vi "PIC1_DEMO.vi"() -> ()   [LabVIEW 2016]
uses:
  <vilib>/picture/picture.llb/imagedata.ctl
panel:
  out "image":u8[](array[numeric]) format="%x"
  out "size(s)":i32[](array[numeric])
  out "24-bit pixmap":u32[][](array[numeric]) format="%x"
  out "image data":T1
  out "new picture":picture
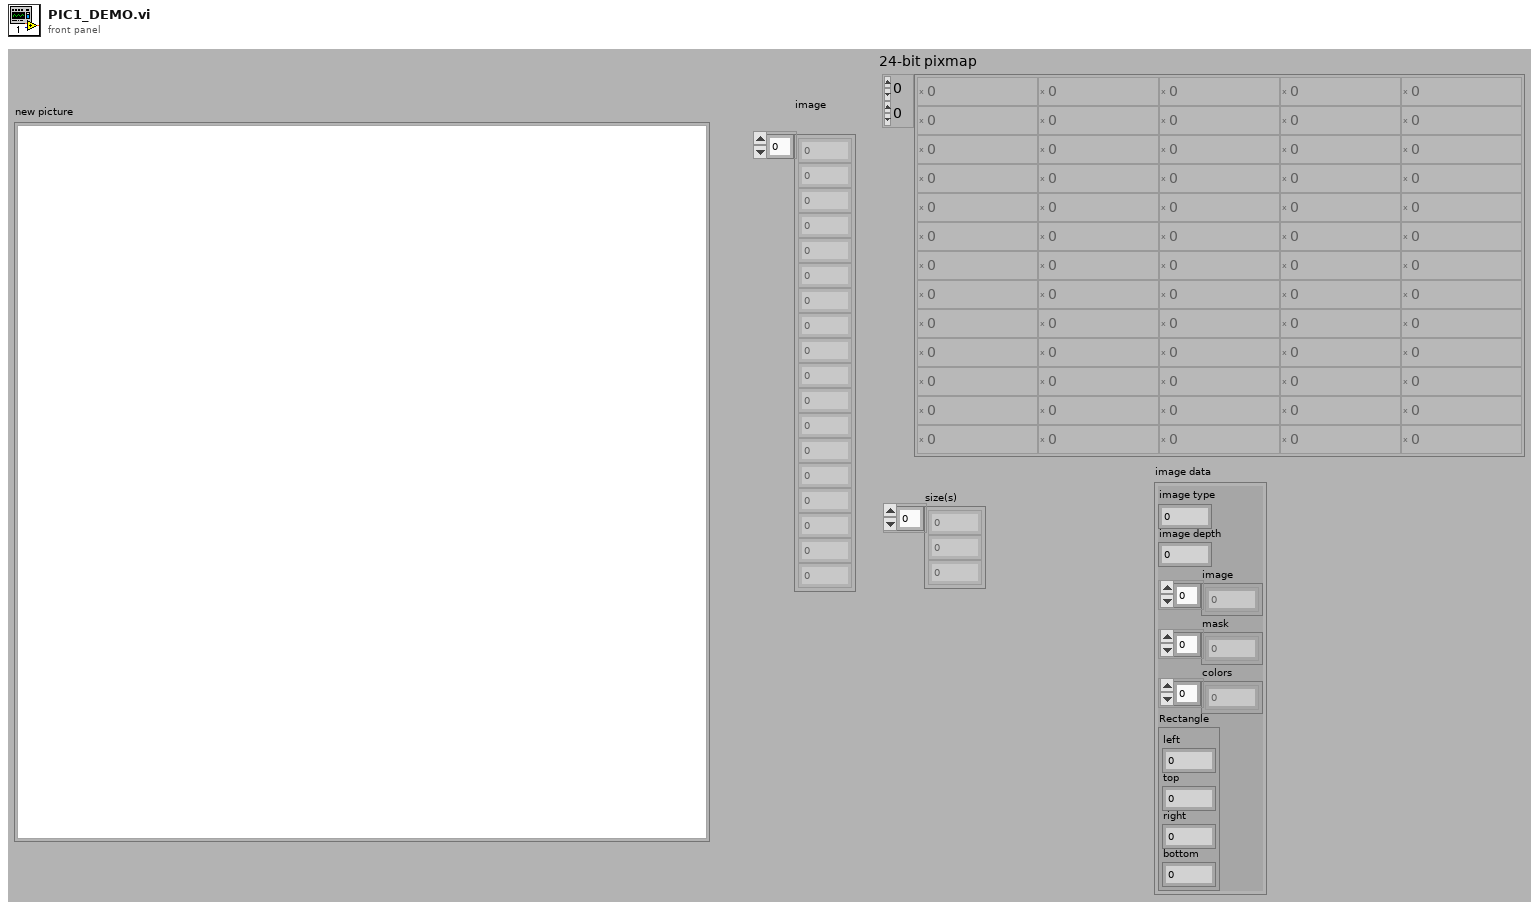
[diagram p1: front panel]
types:
  T1 = typedef "imagedata.ctl" = cluster{"image type":i32, "image depth":i32, "image":u8[], "mask":u8[], "colors":u32[], "Rectangle":cluster{"left":i16, "top":i16, "right":i16, "bottom":i16}}
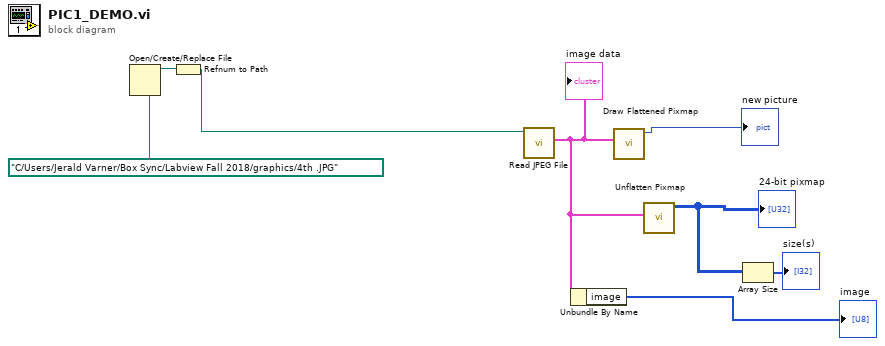
[diagram p0: block diagram]
diagram:
  n1 = Open/Create/Replace File(file path (use dialog)=path "C:/Users/Jerald Varner/Box Sync/Labview Fall 2018/graphics/4th .JPG") -> (refnum out=w5:refnum<file>)  [unwired: 5 in, 2 out]
  n2 = Refnum to Path(1:w5) -> (0:w4:path)
  n3 = call <vilib>:"Read JPEG File.vi"("path to JPEG file"=w4) -> ("image data"=w2:T1)  [unwired: 8 in, 2 out]
  "image data" <- w2
  n4 = Unbundle By Name(w2) -> ("image"=→"image":u8[])
  n5 = call <vilib>:"Draw Flattened Pixmap.vi"("image data"=w2) -> ("new picture"=→"new picture":picture)  [unwired: 8 in]
  n6 = call <vilib>:"Unflatten Pixmap.vi"("image data"=w2) -> ("24-bit pixmap"=w7:u32[][])  [unwired: 4 in, 6 out]
  "24-bit pixmap" <- w7
  n7 = Array Size(array=w7) -> (size(s)=→"size(s)":i32[])
